vi "State_Read Config.vi"(8 "error in (no error)":errorcluster, 11 "launcher in":refnum<class "launcher.lvclass">) -> (0 "error out":errorcluster, 2 "Debug Message":string, 3 "launcher out":refnum<class "launcher.lvclass">)   [LabVIEW 2021, in "launcher.lvclass"]
uses:
  launcher.lvclass
  C:/Program Files (x86)/National Instruments/LabVIEW 2021/user.lib/S2 Labs/Module Framework/Modules/Base/Module.lvclass
  launcher.lvclass/launcher.ctl
  <userlib>/S2 Labs/Module Framework/Modules/Base/Module.lvclass/Module.ctl
  Accessors/_Read Modules to Launch.vi
  <userlib>/S2 Labs/Module Framework/Modules/Base/Write Modules to Launch.vi
  <userlib>/S2 Labs/Module Framework/Modules/Base/Module.lvclass
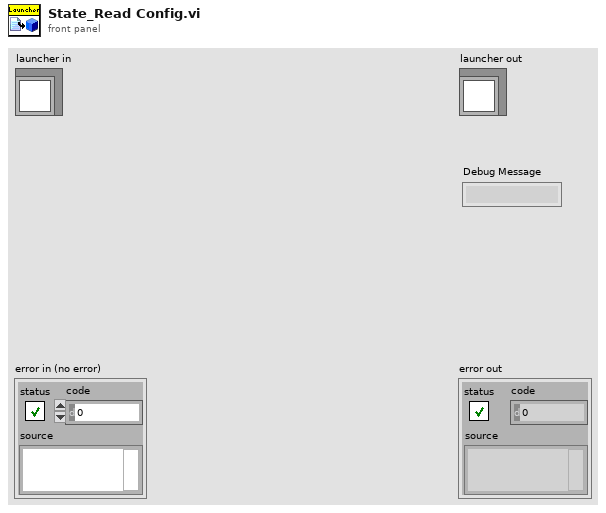
[diagram p1: front panel]
types:
  T1 = typedef "Module.lvclass/Launch Module Typdef.ctl" = cluster{"Module":string, "Parameters":T2}
  T2 = typedef "Module.lvclass/Launch Module Parms.ctl" = cluster{"Name":string, "Arguments":string[], "Show FP?":bool}
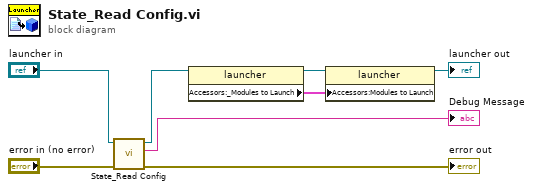
[diagram p0: block diagram]
diagram:
  n1 = call-parent "State_Read Config.vi"("error in (no error)"="error in (no error)", "Module in"="launcher in") -> ("error out"=→"error out":errorcluster, "Debug Message"=→"Debug Message":string, "Module out"=w3:refnum<class "launcher.lvclass">)  [unwired: 7 in]
  n2 = property class="launcher"(reference=w3) -> (reference out=w2:refnum<class "launcher.lvclass">, "Accessors:_Modules to Launch"=w1:T1[])  [unwired: 1 in, 1 out]
  n3 = property class="launcher"(reference=w2, "Accessors:Modules to Launch"=w1) -> (reference out=→"launcher out":refnum<class "launcher.lvclass">)  [unwired: 1 in, 1 out]
